vi "example errors.vi"(11 "timeout?":bool) -> (0 "error out":errorcluster)   [LabVIEW 2011]
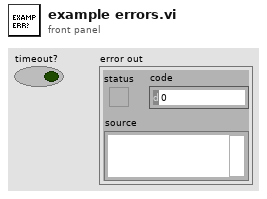
[diagram p1: front panel]
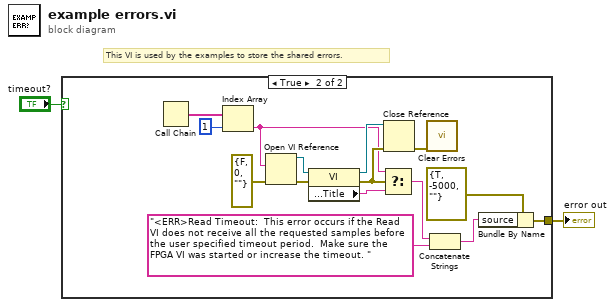
[diagram p0: block diagram]
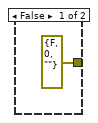
[diagram p2: hidden frame]
diagram:
  # "This VI is used by the examples to store the shared errors."
  n1 = case shown="True" "timeout?" {
    tunnel: [errorcluster {"status"=FALSE, "code"=0, "source"=""} ("error in") w8] -> w2
    frame False {
    }
    frame True {
      n2 = Call Chain() -> (call chain=w14:string[])
      n3 = Index Array(array=w14, index=1) -> (element=w12:string)
      n4 = Open VI Reference(vi path=w12, error in (no error)=errorcluster {"status"=FALSE, "code"=0, "source"=""}) -> (vi reference=w17:refnum<vi>, error out=w16:errorcluster)  [unwired: 4 in]
      n5 = property class="VI"(reference=w17, error in=w16) -> (reference out=w15:refnum<vi>, error out=w13:errorcluster, "Front Panel Window:Title"=w5:string)
      n6 = Select(t=w12, s=w13, f=w5) -> (s? t:f=w4:string)
      n7 = Close Reference(reference=w15, error in (no error)=w13) -> (error out=w6:errorcluster)
      n8 = call <vilib>:"Clear Errors.vi"("error in (no error)"=w6) -> ()  [unwired: 6 in, 1 out]
      n9 = Concatenate Strings(w4, "<ERR>Read Timeout:  This error occurs if the Read VI does not receive all the requested samples before the user specified timeout period.  Make sure the FPGA VI was started or increase the timeout. " ("source")) -> (w9:string)
      n10 = Bundle By Name(cluster=errorcluster {"status"=TRUE, "code"=-5000, "source"=""} ("error out"), "source"=w9) -> (w8:errorcluster)
    }
  }
  "error out" <- w2
